vi "SetupQGStage.vi"() -> ()   [LabVIEW 2009]
uses:
  QGSettings.ctt
panel:
  in  "Cancel Button":bool
  in  "OK Button":bool
  in  "QG Settings":T1={"channels (trigger)"="2", "Trigger Amplitude (V)"=0.1} caption="Stage Setup" {"Trigger Amplitude (V)" format="%.2f"}
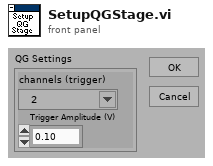
[diagram p1: front panel]
types:
  T1 = typedef "QGSettings.ctt" = cluster{"channels (trigger)":tag, "Trigger Amplitude (V)":dbl}
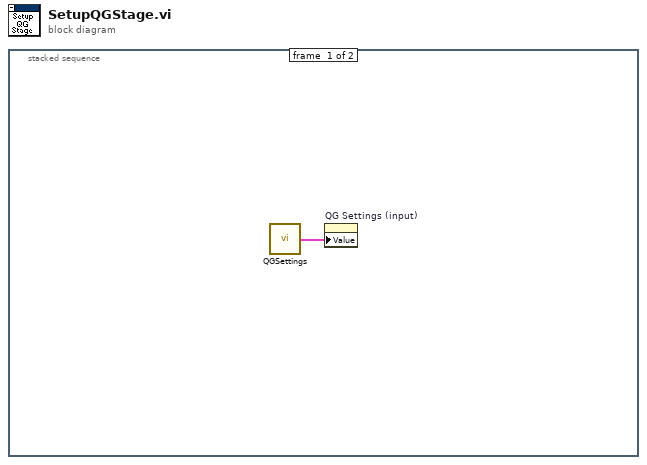
[diagram p0: block diagram]
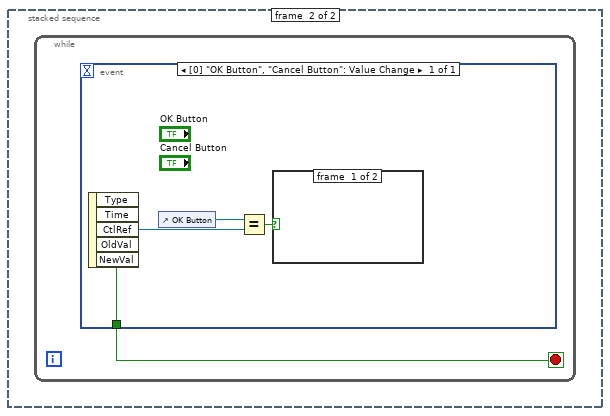
[diagram p2: hidden frame]
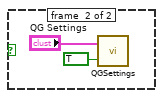
[diagram p3: hidden frame]
diagram:
  n1 = stacked-sequence {
    frame #0 {
      n2 = call "QGSettings.vi"() -> ("QG Settings (output)"=w1:T1)  [unwired: 2 in]
      n3 = property on="QG Settings (input)" class="Clust (strict)"("Value"=w1) -> ()  [unwired: 2 in, 2 out]
    }
    frame #1 {
      n4 = while {
        stop <- w2 stop-if-true
        n5 = event shown="[0] \"OK Button\", \"Cancel Button\": Value Change" {
          selector: _ -> [_]
          dyn-events: _ -> [_]
          timeout: _ -> [_]
          tunnel: [w5] -> w2
          event [0] "OK Button", "Cancel Button": Value Change {
            n6 = event-data() -> ("CtlRef"=w6:refnum<vi>, "NewVal"=w5:bool)  [unwired: 1 in, 3 out]
            n7 = control-ref of="OK Button"() -> (w3:refnum<vi>)
            n8 = Equal?(x=w3, y=w6) -> (x = y?=w4:bool)
            n9 = case shown="True" w4 {
              frame #0 {
              }
              frame #1 {
                n10 = call "QGSettings.vi"("Set/Get"=TRUE ("Get/Set"), "QG Settings (input)"="QG Settings") -> ()  [unwired: 1 out]
              }
            }
          }
        }
      }
    }
  }
